vi "UserComment.vi"(5 "EndTime":timestamp, 7 "StartTime":timestamp, 8 "error in":errorcluster, 11 "UserComment":refnum<class "UserComment.lvclass">) -> (0 "error out":errorcluster, 3 "Passed":bool)   [LabVIEW 2020]
uses:
  ProligentResultProcessor/Model/UserComment/UserComment.lvclass
  ProligentResultProcessor/Model/UserComment/SetComment.vi
  ProligentResultProcessor/Model/UserComment/SetTime.vi
  ProligentResultProcessor/Model/UserComment/SetUser.vi
  ProligentResultProcessor/Model/UserComment/GetComment.vi
  ProligentResultProcessor/Model/UserComment/GetTime.vi
  ProligentResultProcessor/Model/UserComment/GetUser.vi
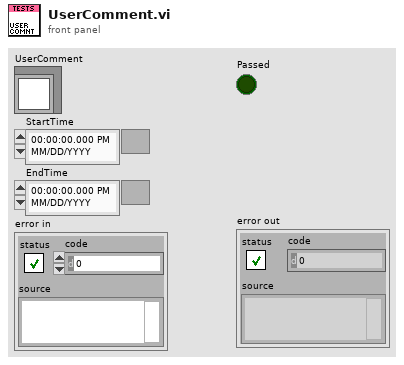
[diagram p1: front panel]
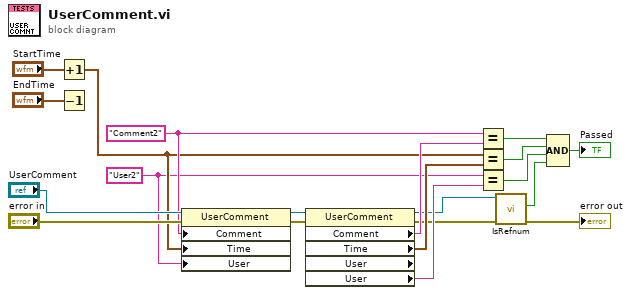
[diagram p0: block diagram]
diagram:
  w1 = "User2"
  w13 = "Comment2"
  n1 = Increment(x="StartTime") -> (x+1=w2:timestamp)
  n2 = Decrement(x="EndTime") -> ()  [unwired: 1 out]
  n3 = property class="UserComment"(reference="UserComment", error in="error in", "Comment"=w13, "Time"=w2, "User"=w1) -> (reference out=w18:refnum<class "UserComment.lvclass">, error out=w17:errorcluster)
  n4 = property class="UserComment" props=["Comment", "Time", "User", "User"](reference=w18, error in=w17) -> (reference out=w3:refnum<class "UserComment.lvclass">, error out=w12:errorcluster, "Comment"=w16:string, "Time"=w15:timestamp, "User"=w14:string)  [unwired: 1 out]
  n5 = Equal?(x=w13, y=w16) -> (x = y?=w11:bool)
  n6 = Equal?(x=w2, y=w15) -> (x = y?=w10:bool)
  n7 = Equal?(x=w1, y=w14) -> (x = y?=w9:bool)
  n8 = call "IsRefnum.vi"("error in"=w12, "UserComment in"=w3) -> ("error out"=→"error out":errorcluster, "IsRefnum"=w4:bool)  [unwired: 7 in, 1 out]
  n9 = Compound Arithmetic op=AND(w11, w10, w9, w4) -> (→"Passed":bool)
